vi "GetInput1.vi"() -> (0 "Buttons":bool[](array[boolean]), 3 "Axes":dbl[](array[numeric]))   [LabVIEW 2020]
uses:
  <vilib>/Rock Robotics/WPI/Utilities/WPI_GetSetVariantRefNum.vi
  <vilib>/Rock Robotics/Network Tables/NT Write Boolean Array.vi
  <vilib>/Rock Robotics/Network Tables/NT Write Numeric Array.vi
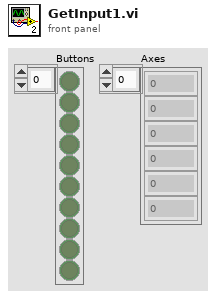
[diagram p1: front panel]
types:
  T1 = typedef "WPI_JoystickDevRef.ctl" = cluster{"Device":T2}
  T2 = typedef "WPI_JoystickDeviceEnum.ctl" = enum16{"USB 0", "USB 1", "USB 2", "USB 3", "USB 4", "USB 5"}
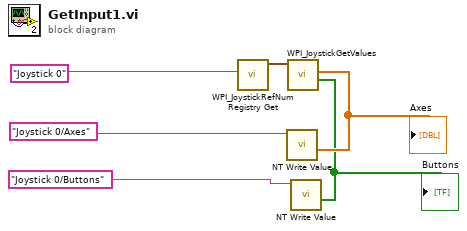
[diagram p0: block diagram]
diagram:
  n1 = call <vilib>:"WPI_JoystickRefNum Registry Get.vi"("refnum name"="Joystick 0") -> ("JoystickDevRef"=w5:T1)  [unwired: 1 in, 9 out]
  n2 = call <vilib>:"WPI_JoystickGetValues.vi"("JoystickDevRef"=w5) -> ("Buttons"=w1:bool[], "Axes"=w2:dbl[])  [unwired: 6 in, 3 out]
  "Buttons" <- w1
  "Axes" <- w2
  n3 = call-poly <vilib>:"NT Write Value.vi"("Numeric Array"=w2, "Name"="Joystick 0/Axes") -> ()  [unwired: 9 in, 1 out]
  n4 = call-poly <vilib>:"NT Write Value.vi"("Boolean Array"=w1, "Name"="Joystick 0/Buttons") -> ()  [unwired: 9 in, 1 out]
